vi "QueryHealthAndStatus.vi"(11 "HealthAndStatusSettings":T1={"InternalHealthAndStatusFIFO"="InternalTelemetryFIFO", "HealthAndStatusQueryFIFO"="TelemetryQueryFIFO", "HealthAndStatusResponseFIFO"="TelemetryResponseFIFO", "HealthAndStatusMemory"="TelemetryMemory", "MemorySize"=0}) -> ()   [LabVIEW 2015, in "FPGAHealthAndStatus.lvlib"]
uses:
  FPGAHealthAndStatus.lvlib
  <vilib>/rvi/DataTransferAndStorage/Container/XNode/niFpgaContainer.xnode
  DataTypes/QueryHealthAndStatusStates.ctl
  DataTypes/QueryHealthAndStatusLoopData.ctl
  <vilib>/rvi/FIFO/Fifo_Resource/niFpgaFifoEmulationRefIn.vi
  <vilib>/rvi/Memory/Memory_Emulation/niFpgaMemoryEmulationRefIn.vi
  DataTypes/HealthAndStatusSettings.ctl
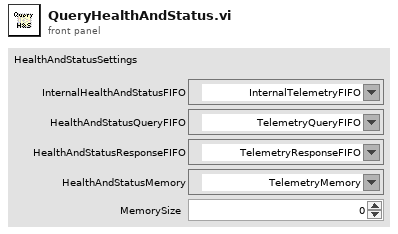
[diagram p1: front panel]
types:
  T1 = typedef "FPGAHealthAndStatus.lvlib/HealthAndStatusSettings.ctl" = cluster{"InternalHealthAndStatusFIFO":refnum<k21>, "HealthAndStatusQueryFIFO":refnum<k21>, "HealthAndStatusResponseFIFO":refnum<k21>, "HealthAndStatusMemory":refnum<k21>, "MemorySize":i32}
  T2 = typedef "FPGAHealthAndStatus.lvlib/QueryHealthAndStatusLoopData.ctl" = cluster{"State":T3, "InstructionData":u32, "AddressOffset":u32}
  T3 = typedef "FPGAHealthAndStatus.lvlib/QueryHealthAndStatusStates.ctl" = enum16{"Try Read Instruction", "Send Telemetry", "Send All Telemetry"}
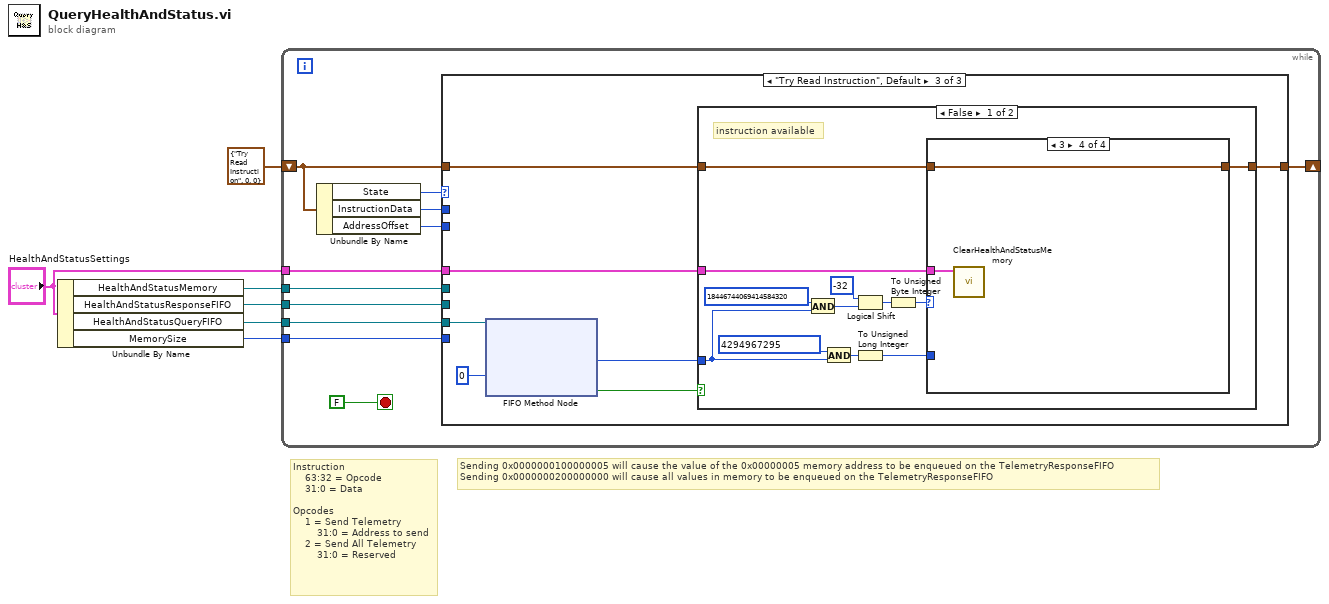
[diagram p0: block diagram]
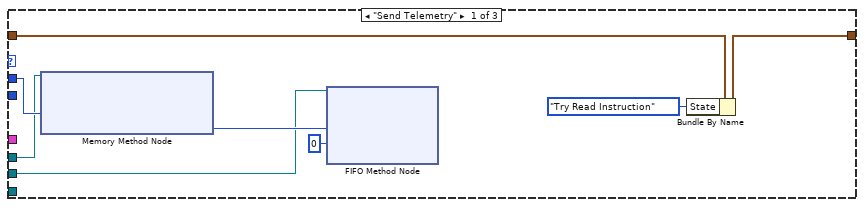
[diagram p2: hidden frame]
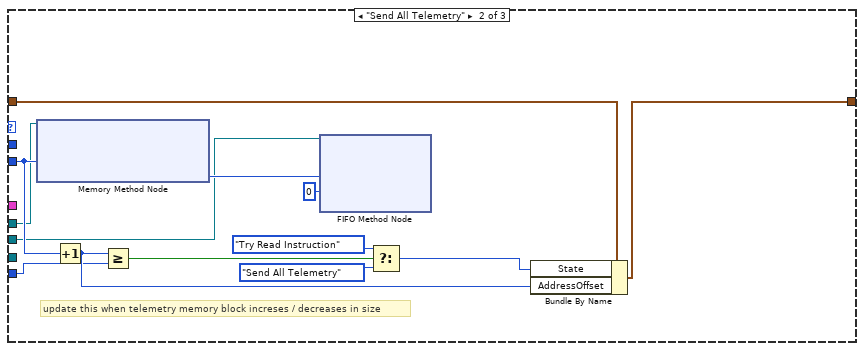
[diagram p3: hidden frame]
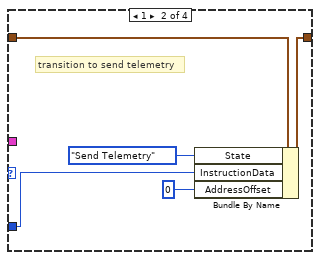
[diagram p5: hidden frame]
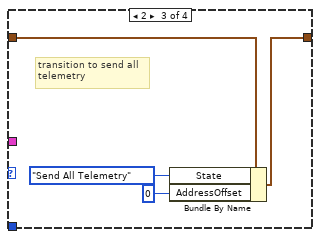
[diagram p6: hidden frame]
diagram:
  # "Sending 0x0000000100000005 will cause the value of the 0x00000005 memory address to be enqueued on the TelemetryResponseFIFO\nSending 0x0000000200000000 will cause all values in memory to be enqueued on the TelemetryResponseFIFO"
  # "Instruction\n    63:32 = Opcode\n    31:0 = Data\n\nOpcodes\n    1 = Send Telemetry\n        31:0 = Address to send\n    2 = Send All Telemetry\n        31:0 = Reserved"
  n1 = Unbundle By Name("HealthAndStatusSettings") -> ("HealthAndStatusMemory"=w2:refnum<k21>, "HealthAndStatusResponseFIFO"=w3:refnum<k21>, "HealthAndStatusQueryFIFO"=w4:refnum<k21>, "MemorySize"=w5:i32)
  n2 = while {
    shift-right: [w14] -> _
    shift-left: T2 {"State"=enum."Try Read Instruction", "InstructionData"=0, "AddressOffset"=0} ("Command Telemetry Loop") -> [w16]
    tunnel: w4 -> [w11]
    tunnel: w2 -> [w10]
    tunnel: w3 -> [w9]
    tunnel: w5 -> [w8]
    tunnel: "HealthAndStatusSettings" -> [w7]
    stop <- FALSE stop-if-true
    n3 = Unbundle By Name(w16) -> ("State"=w17:T3, "InstructionData"=w15:u32, "AddressOffset"=w13:u32)
    n4 = case shown="\"Try Read Instruction\", Default" w17 {
      tunnel: w16 -> [w25 w38 w44]
      tunnel: w15 -> [w23 _ _]
      tunnel: [w24 w37 w43] -> w14
      tunnel: w13 -> [_ w34 _]
      tunnel: w11 -> [_ _ w40]
      tunnel: w10 -> [w19 w28 _]
      tunnel: w9 -> [w18 w27 _]
      tunnel: w8 -> [_ w26 _]
      tunnel: w7 -> [_ _ w39]
      frame "Send Telemetry" {
        n5 = xnode ("Memory Method Node")("Address"=w23, "Memory In"=w19) -> ("Data"=w21:u32)  [unwired: 1 out]
        n6 = xnode ("FIFO Method Node")("Element"=w21, "Timeout"=0, "FIFO In"=w18) -> ()  [unwired: 2 out]
        n7 = Bundle By Name(cluster=w25, "State"=QueryHealthAndStatusStates."Try Read Instruction" ("f")) -> (w24:T2)
      }
      frame "Send All Telemetry" {
        # "update this when telemetry memory block increses / decreases in size"
        n8 = xnode ("Memory Method Node")("Address"=w34, "Memory In"=w28) -> ("Data"=w36:u32)  [unwired: 1 out]
        n9 = Increment(x=w34) -> (x+1=w29:u32)
        n10 = Greater Or Equal?(x=w29, y=w26) -> (x >= y?=w33:bool)
        n11 = xnode ("FIFO Method Node")("Element"=w36, "Timeout"=0, "FIFO In"=w27) -> ()  [unwired: 2 out]
        n12 = Select(t=QueryHealthAndStatusStates."Try Read Instruction" ("f"), s=w33, f=QueryHealthAndStatusStates."Send All Telemetry") -> (s? t:f=w30:T3)
        n13 = Bundle By Name(cluster=w38, "State"=w30, "AddressOffset"=w29) -> (w37:T2)
      }
      frame "Try Read Instruction", Default {
        n14 = xnode ("FIFO Method Node")("Timeout"=0, "FIFO In"=w40) -> ("Element"=w45:u64, "Timed Out?"=w41:bool)  [unwired: 1 out]
        n15 = case shown="False" w41 {
          tunnel: w45 -> [w47 _]
          tunnel: w44 -> [w57 w70]
          tunnel: [w56 w70] -> w43
          tunnel: w39 -> [w46 _]
          frame False {
            # "instruction available"
            n16 = And(x=u64 18446744069414584320, y=w47) -> (x .and. y?=w53:u64)
            n17 = And(x=u64 4294967295, y=w47) -> (x .and. y?=w49:u64)
            n18 = Logical Shift(y=i16 -32, x=w53) -> (x << y=w51:u64)
            n19 = To Unsigned Long Integer(number=w49) -> (unsigned 32bit integer=w48:u32)
            n20 = To Unsigned Byte Integer(number=w51) -> (unsigned 8bit integer=w50:u8)
            n21 = case shown="3" w50 {
              tunnel: w57 -> [w58 w63 w67 w69]
              tunnel: [w58 w62 w66 w69] -> w56
              tunnel: w48 -> [_ w59 _ _]
              tunnel: w46 -> [_ _ _ w68]
              frame 0, Default {
                # "nop"
              }
              frame 1 {
                # "transition to send telemetry"
                n22 = Bundle By Name(cluster=w63, "State"=QueryHealthAndStatusStates."Send Telemetry", "InstructionData"=w59, "AddressOffset"=u32 0 ("Telemetry Offset")) -> (w62:T2)
              }
              frame 2 {
                # "transition to send all \ntelemetry"
                n23 = Bundle By Name(cluster=w67, "State"=QueryHealthAndStatusStates."Send All Telemetry", "AddressOffset"=u32 0 ("Telemetry Offset")) -> (w66:T2)
              }
              frame 3 {
                n24 = call "ClearHealthAndStatusMemory.vi"("HealthAndStatusSettings"=w68) -> ()  [unwired: 11 in]
              }
            }
          }
          frame True {
            # "no instruction available"
          }
        }
      }
    }
  }
